vi "FlowChart String Analize.vi"(8 "error in (no error)":errorcluster caption="Error In", 10 "Old Value":variant, 11 "New Value":variant) -> (0 "error out":errorcluster caption="Error Out", 2 "Set":cluster{"Name":string, "Data":string}, 3 "Data":cluster{"Index":i32, "Data":variant})   [LabVIEW 2020]
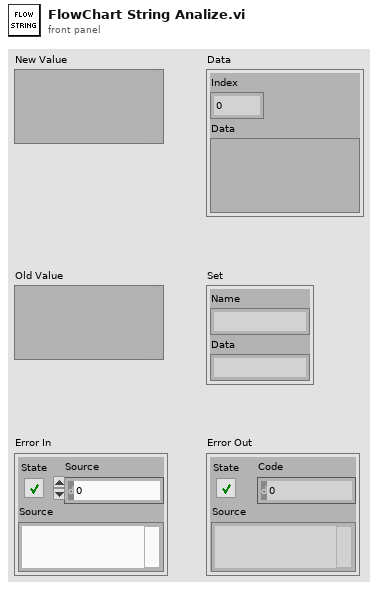
[diagram p1: front panel]
types:
  T1 = cluster{cluster{"String":string, "String":string}[]}
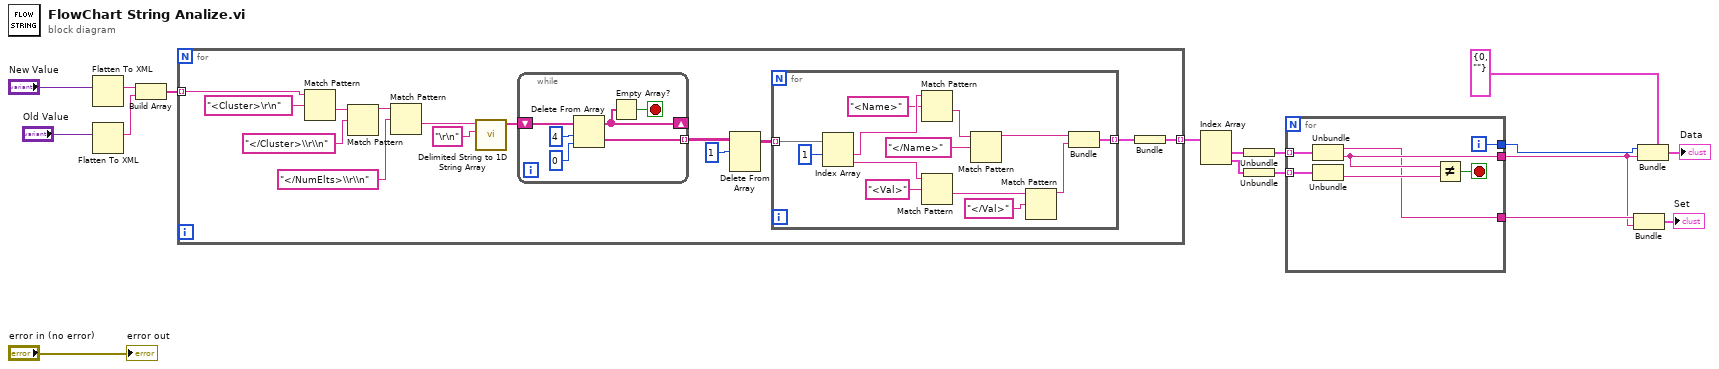
[diagram p0: block diagram]
diagram:
  n1 = Flatten To XML(6:"New Value") -> (2:w15:string)
  n2 = Flatten To XML(6:"Old Value") -> (2:w14:string)
  n3 = Build Array(w15, w14) -> (w13:string[])
  n4 = for {
    tunnel: w13 -> [w20] mode=indexing
    tunnel: [w18] -> w12 mode=indexing
    n5 = Match Pattern(string=w20, regular expression="<Cluster>\r\n" ("正则表达式")) -> (after substring=w30:string)  [unwired: 1 in, 3 out]
    n6 = Match Pattern(string=w30, regular expression="</Cluster>\\r\\n" ("正则表达式")) -> (before substring=w28:string)  [unwired: 1 in, 3 out]
    n7 = Match Pattern(string=w28, regular expression="</NumElts>\\r\\n" ("正则表达式")) -> (after substring=w26:string)  [unwired: 1 in, 3 out]
    n8 = call <vilib>:"Delimited String to 1D String Array.vi"("delimiter"="\r\n", "delimited string"=w26) -> ("string array"=w24:string[])  [unwired: 9 in]
    n9 = while {
      shift-right: [w46] -> _
      shift-left: w24 -> [w50]
      tunnel: [w45] -> w23 mode=indexing
      stop <- w49 stop-if-true
      n10 = Delete From Array(array=w50, length=4 ("长度"), index=0 ("索引")) -> (deleted portion=w45:string[], array with subset deleted=w46:string[])
      n11 = Empty Array?(array=w46) -> (empty?=w49:bool)
    }
    n12 = Delete From Array(array=w23, length=1 ("长度")) -> (array with subset deleted=w21:string[][])  [unwired: 2 in, 1 out]
    n13 = for {
      tunnel: w21 -> [w44] mode=indexing
      tunnel: [w32] -> w19 mode=indexing
      n14 = Index Array(array=w44, index #1=1 ("索引")) -> (element #1=w41:string, element #2=w37:string)  [unwired: 1 in]
      n15 = Match Pattern(string=w41, regular expression="<Name>" ("正则表达式")) -> (after substring=w42:string)  [unwired: 1 in, 3 out]
      n16 = Match Pattern(string=w37, regular expression="<Val>" ("正则表达式")) -> (after substring=w38:string)  [unwired: 1 in, 3 out]
      n17 = Match Pattern(string=w42, regular expression="</Name>" ("正则表达式")) -> (before substring=w34:string)  [unwired: 1 in, 3 out]
      n18 = Match Pattern(string=w38, regular expression="</Val>" ("正则表达式")) -> (before substring=w33:string)  [unwired: 1 in, 3 out]
      n19 = Bundle("String"=w34, "String"=w33) -> (w32:cluster{"String":string, "String":string})  [unwired: 1 in]
    }
    n20 = Bundle(w19) -> (w18:T1)  [unwired: 1 in]
  }
  n21 = Index Array(array=w12) -> (element #1=w11:T1, element #2=w10:T1)  [unwired: 2 in]
  n22 = Unbundle(w11) -> (w9:cluster{"String":string, "String":string}[])
  n23 = Unbundle(w10) -> (w8:cluster{"String":string, "String":string}[])
  n24 = for {
    tunnel: w9 -> [w57] mode=indexing
    tunnel: w8 -> [w56] mode=indexing
    tunnel: [w54] -> w7
    tunnel: [w52] -> w2
    tunnel: [w51] -> w3
    i -> [w54]
    stop <- w55 stop-if-true
    n25 = Unbundle(w57) -> ("String"=w51:string, "String"=w52:string)
    n26 = Unbundle(w56) -> ("String"=w53:string)  [unwired: 1 out]
    n27 = Not Equal?(x=w52, y=w53) -> (x != y?=w55:bool)
  }
  n28 = Bundle("String"=w3, "String"=w2) -> (→"Set":cluster{"String":string, "String":string})  [unwired: 1 in]
  n29 = Bundle(cluster=cluster{i32, "Value":string} {0, "Value"=""}, w7, "Value"=w2) -> (→"Data":cluster{i32, "Value":string})
  "error out" <- "error in (no error)"
